vi "NumeroAureo.vi"() -> (0 "Numero aureo":dbl format="%.18f")   [LabVIEW 2022 SP3]
doc: "Calcula el número áureo de la forma: (sqrt(5)+1)/2"
panel:
  # "Numero Aureo"
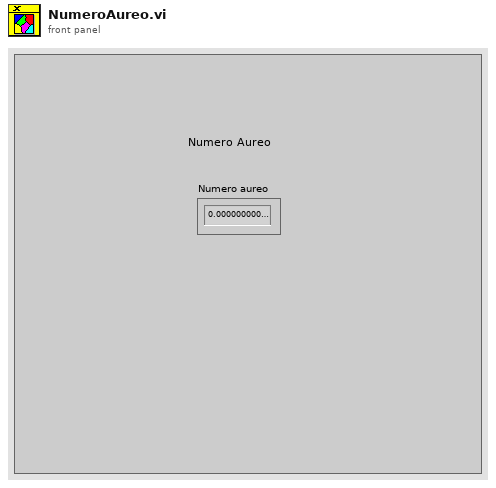
[diagram p1: front panel]
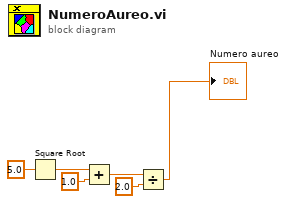
[diagram p0: block diagram]
diagram:
  n1 = Square Root(x=5.0) -> (sqrt(x)=w4:dbl)
  n2 = Add(x=w4, y=1.0) -> (x+y=w5:dbl)
  n3 = Divide(x=w5, y=2.0) -> (x/y=→"Numero aureo":dbl)
